vi "OFBS_MainFunction.vi"(6 "ReInitialize?":bool, 8 "Stop ButtonRef in":refnum<vi>, 9 "Results ListBox Ref":refnum<vi>, 10 "Fitness Chart Ref in":refnum<vi>, 11 "OFBS metaparameters in":T1={"Training Data Path"=path "", "Test Data Path"=path "", "True Labels for Test Trials"=path "", "Optimization Algorithm"=enum."Genetic algorithm", "ClassifierType"=enum."Multilayer perceptron", "GA Parameters"={"Population size"=100, "Generations no."=500, "Significant digits"=4, "Crossover probabality"=0.85, "Mutation mode"=enum."one-point, fixed rate", "Use Gray code?"=FALSE, "Mutation rate"=0.05, "Min mutation rate"=0.0005, "Max mutation rate"=0.25, "Reproduction plan"=enum."Steady-state-replace-worst", "Elitism"=FALSE, "Fmax"=1}, "PSO Parameters"={"Swarm size"=50, "Generations no."=10, "Cognitive coeff a1"=2.05, "Social coeff a2"=2.05, "Min inertia weight"=0.4, "Max inertia weight "=0.9, "Fmax"=0}, "Number of Channels"=0, "Use equal number of trials?"=FALSE, "Classifier Metaparameter"=0.0, "ClassifierQualityMeasure"=enum."Accuracy"} {"Classifier Metaparameter" min=0.0 max=100.0 step=0.1 format="%#_2g"; "PSO Parameters"."Generations no." min=1; "PSO Parameters"."Swarm size" min=1; "GA Parameters"."Max mutation rate" min=0.0 max=1.0; "GA Parameters"."Min mutation rate" min=0.0 max=1.0; "GA Parameters"."Mutation rate" min=0.0 max=1.0; "GA Parameters"."Crossover probabality" min=0.0 max=1.0; "GA Parameters"."Significant digits" min=1; "GA Parameters"."Generations no." min=1; "GA Parameters"."Population size" min=1}) -> (0 "Results dbl":dbl[](array[numeric]), 3 "Results str":string[](array[string]))   [LabVIEW 2016, in "Optimal Frequency Bands Search.lvlib"]
doc: "Главный виртуальный прибор проекта. Реализует графический интерфейс взаимодействия с пользователем."
uses:
  Optimal Frequency Bands Search.lvlib
  _vlib/OFBS_metaParameters.ctl
  _vlib/OFBS_AlgorithmTypes.ctl
  4. Accuracy Assessment for EEG Classification/_vlib/CU_ClassifierTypes.ctl
  GA_core/GA_tParameters.ctl
  particle_swarm_opt/PSO_tParameters.ctl
  4. Accuracy Assessment for EEG Classification/_vlib/CU_ClassifierQualityMeasure.ctl
  _vlib/OFBS_AppStates.ctl
  _vlib/OptFreqBandsSearch.lvclass
  GA_core/GA_tFitness Function.ctl
  GA_core/GA_tPopulation.ctl
  GA_core/GA_tSolution progress.ctl
  particle_swarm_opt/tFitness Function.ctl
  particle_swarm_opt/PSO_tPopulation.ctl
  particle_swarm_opt/PSO_tSolution progress.ctl
  GA_core/GeneticAlgorithm.lvlib
  particle_swarm_opt/ParticleSwarm.lvlib
  4. Accuracy Assessment for EEG Classification/Classifier.lvlib
panel:
  out "Solution":i32[][][](array[numeric])
  out "Accuracy":dbl caption="Приспособ-\nленность"
  out "Generation":i32 caption="Поколение"
  out "Trials of each class":i32[](array[numeric]) caption="Число проб \nкаждого класса"
  out "Reading File":path caption="Чтение файла"
  out "Progress":i32(slide) caption="Процесс чтения" min=0 max=320 scale=0.0..288.0
  out "Number of Trials":i32 caption="Число проб в файле"
  out "Application State":string caption="Состояние"
  # "This VI is a part of BCI Design library, http://www.ru-bci.org \nCopyright © 2020, Sotnikov Peter, All rights reserved. License: CC BY-NC 4.0"
  # "Fo"
  # "deltaF"
  # "Точность\nна тестовой\nвыборке"
  # "Точность\nна обучающей\nвыборке"
  # "Точность\nна контрол. \nвыборке"
  # "Sotnikov P (c), 2016"
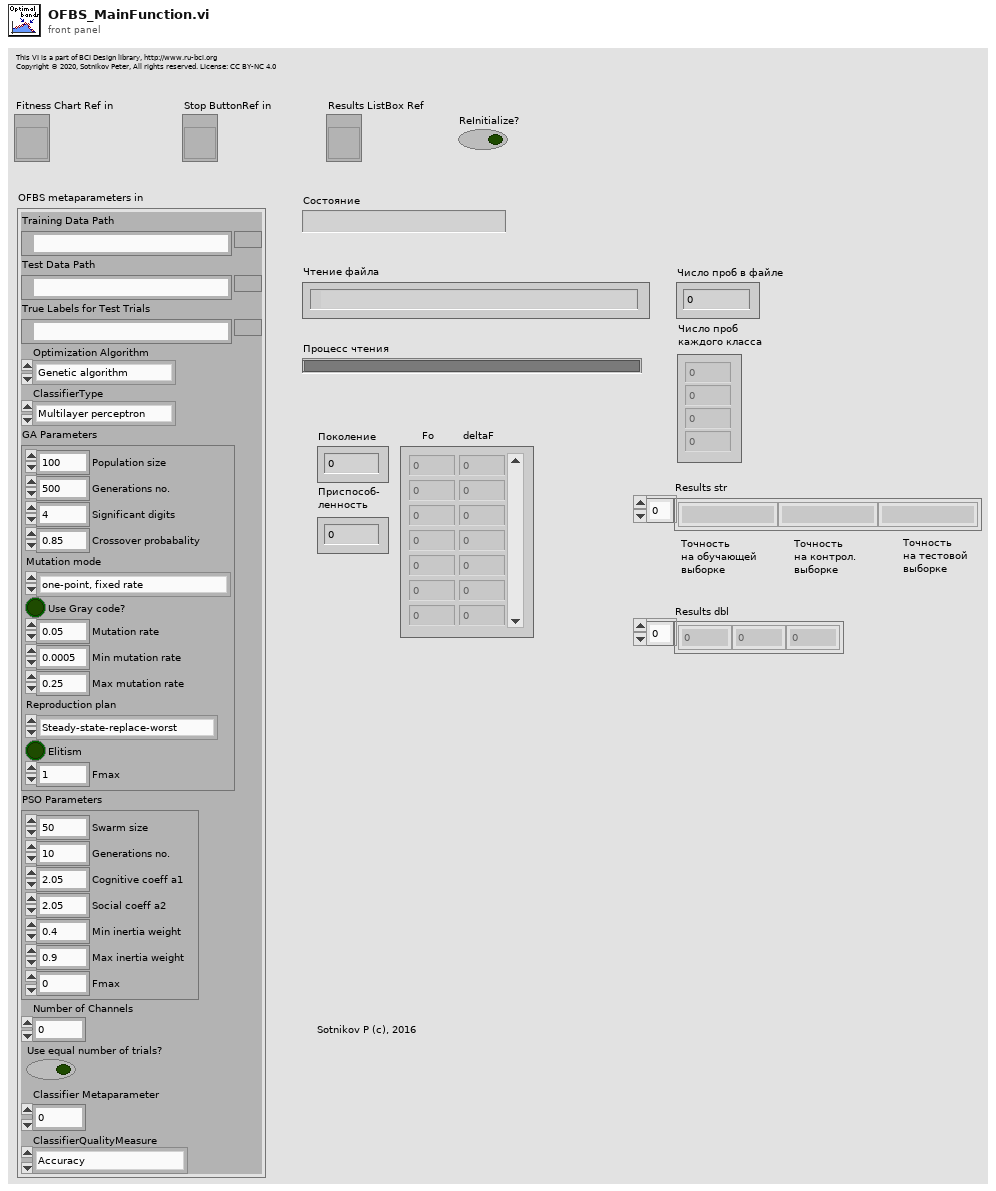
[diagram p1: front panel]
types:
  T1 = typedef "Optimal Frequency Bands Search.lvlib/OFBS_metaParameters.ctl" = cluster{"Training Data Path":path, "Test Data Path":path, "True Labels for Test Trials":path, "Optimization Algorithm":T2, "ClassifierType":T3, "GA Parameters":T4, "PSO Parameters":T5, "Number of Channels":i32, "Use equal number of trials?":bool, "Classifier Metaparameter":dbl, "ClassifierQualityMeasure":T6}
  T2 = typedef "Optimal Frequency Bands Search.lvlib/OFBS_AlgorithmTypes.ctl" = enum16{"Genetic algorithm", "Particle swarm optimization"}
  T3 = typedef "Classifier.lvlib/CU_ClassifierTypes.ctl" = enum16{"Multilayer perceptron", "k NN Classifier", "SVM Committee", "Mahalanobis distance", "SVM Classifier"}
  T4 = typedef "Optimal Frequency Bands Search.lvlib/GeneticAlgorithm.lvlib/GA_tParameters.ctl" = cluster{"Population size":i32, "Generations no.":i32, "Significant digits":i32, "Crossover probabality":dbl, "Mutation mode":enum16{"one-point, fixed rate", "one-point, fitness-adjustable rate", "one-point, distance-adjustable rate"}, "Use Gray code?":bool, "Mutation rate":dbl, "Min mutation rate":dbl, "Max mutation rate":dbl, "Reproduction plan":enum16{"Full generational replacement", "Steady-state-replace-random", "Steady-state-replace-worst"}, "Elitism":bool, "Fmax":i32}
  T5 = typedef "Optimal Frequency Bands Search.lvlib/ParticleSwarm.lvlib/PSO_tParameters.ctl" = cluster{"Swarm size":i32, "Generations no.":i32, "Cognitive coeff a1":dbl, "Social coeff a2":dbl, "Min inertia weight":dbl, "Max inertia weight ":dbl, "Fmax":i32}
  T6 = typedef "Classifier.lvlib/CU_ClassifierQualityMeasure.ctl" = enum16{"Accuracy", "Cohen's kappa"}
  T7 = typedef "Optimal Frequency Bands Search.lvlib/OFBS_AppStates.ctl" = enum16{"Initialize", "ReadTrainData", "ReadTestData", "StartOptimization", "Optimization_GA", "Optimization_PSO", "Stop"}
  T8 = typedef "Optimal Frequency Bands Search.lvlib/GeneticAlgorithm.lvlib/GA_tFitness Function.ctl" = refnum<vi>
  T9 = typedef "Optimal Frequency Bands Search.lvlib/ParticleSwarm.lvlib/tFitness Function.ctl" = refnum<vi>
  T10 = cluster{"Training Data Path":path, "Test Data Path":path, "True Labels for Test Trials":path}
  T11 = cluster{"Number of Trials":refnum<vi>, "Progress":refnum<vi>}
  T12 = typedef "Optimal Frequency Bands Search.lvlib/GeneticAlgorithm.lvlib/GA_tSolution progress.ctl" = cluster{"Solution":i32[], "Fitness":dbl, "Mutation rate":dbl, "Generation":i32}
  T13 = typedef "Optimal Frequency Bands Search.lvlib/GeneticAlgorithm.lvlib/GA_tPopulation.ctl" = cluster{"Population":i32[][], "Fitnesses":dbl[], "Sorted indices":i32[], "Ranks":i32[]}
  T14 = cluster{"Accuracy":refnum<vi>, "Generation":refnum<vi>, "Solution":refnum<vi>, "Fitness Chart Ref in":refnum<vi>}
  T15 = typedef "Optimal Frequency Bands Search.lvlib/ParticleSwarm.lvlib/PSO_tSolution progress.ctl" = cluster{"Solution":i32[], "Fitness":dbl, "Inertia":dbl, "Generation":i32}
  T16 = typedef "Optimal Frequency Bands Search.lvlib/ParticleSwarm.lvlib/PSO_tPopulation.ctl" = cluster{"Particle Coordinates":i32[][], "Fitnesses":dbl[], "Sorted indices":i32[], "Pbest Fitnesses":dbl[], "Pbest Particle Coordinates":i32[][], "Previous Velocity":dbl[][]}
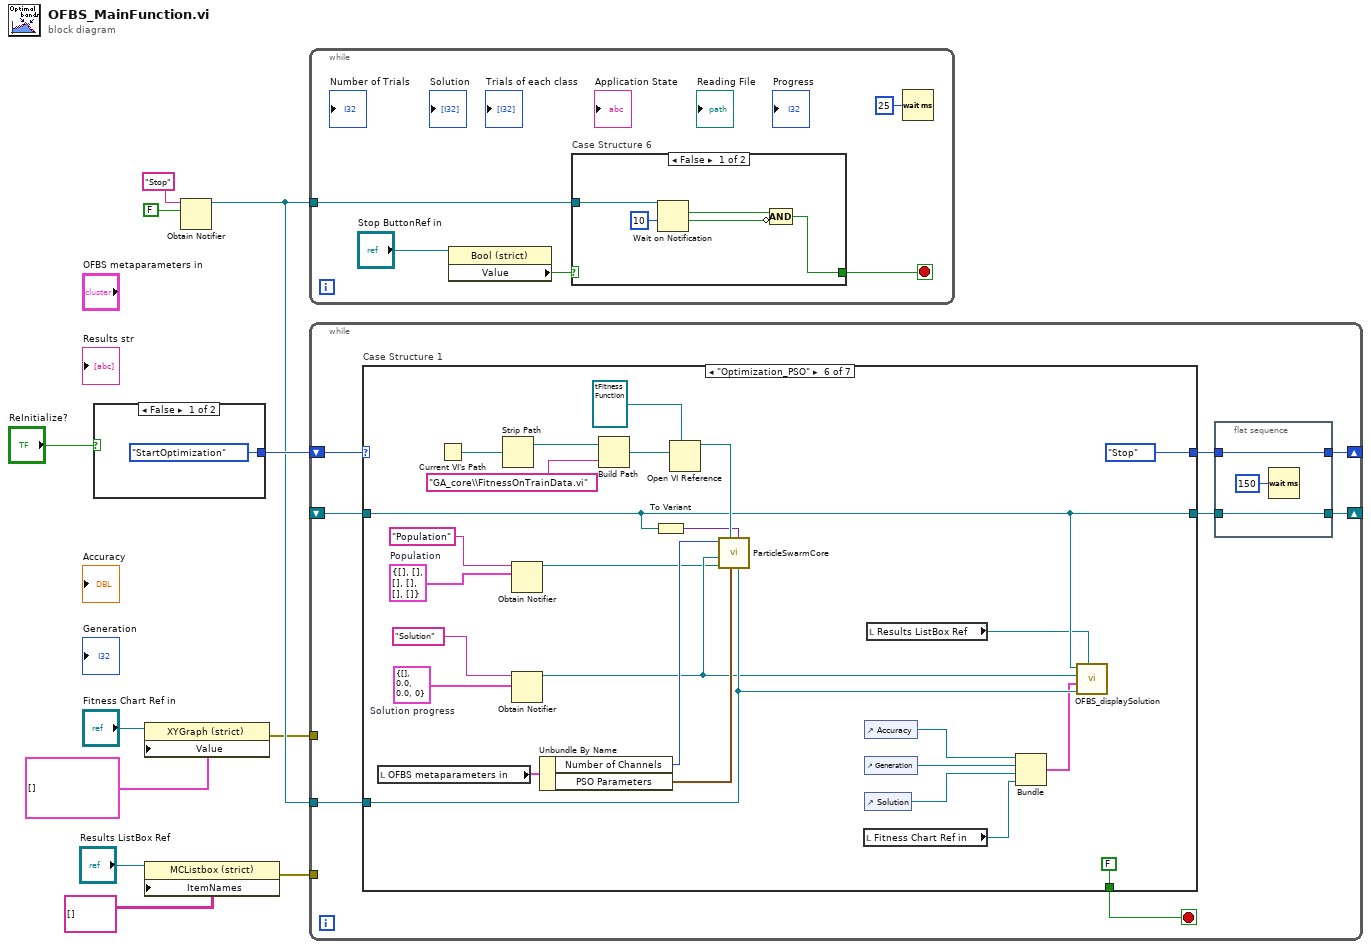
[diagram p0: block diagram]
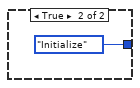
[diagram p2: hidden frame]
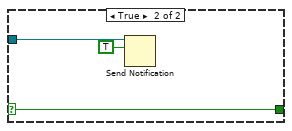
[diagram p3: hidden frame]
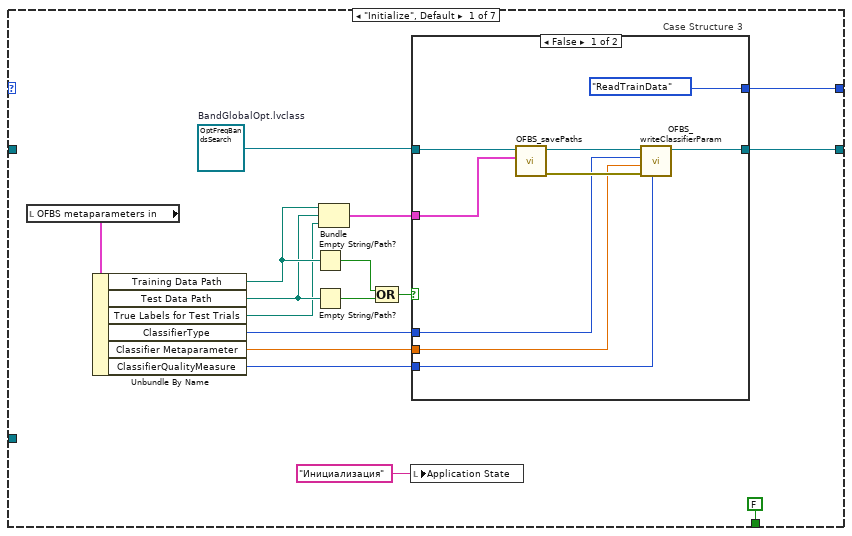
[diagram p4: hidden frame]
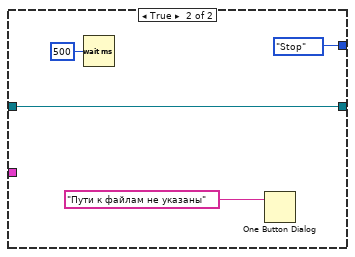
[diagram p5: hidden frame]
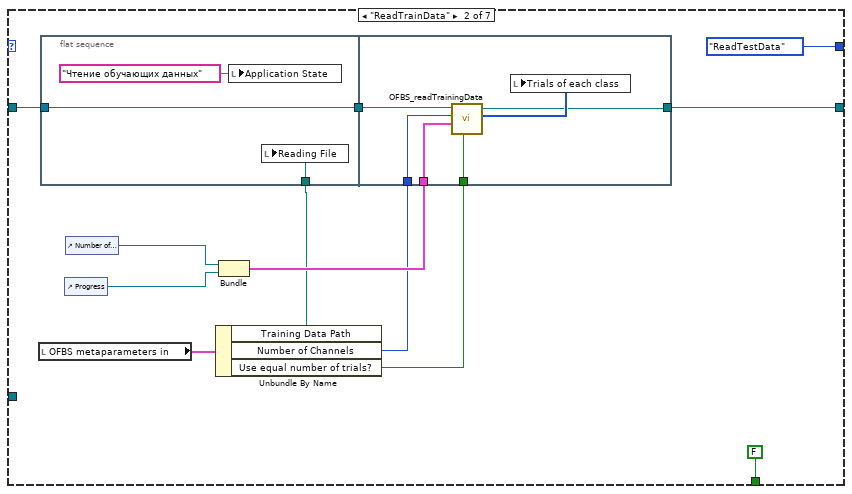
[diagram p6: hidden frame]
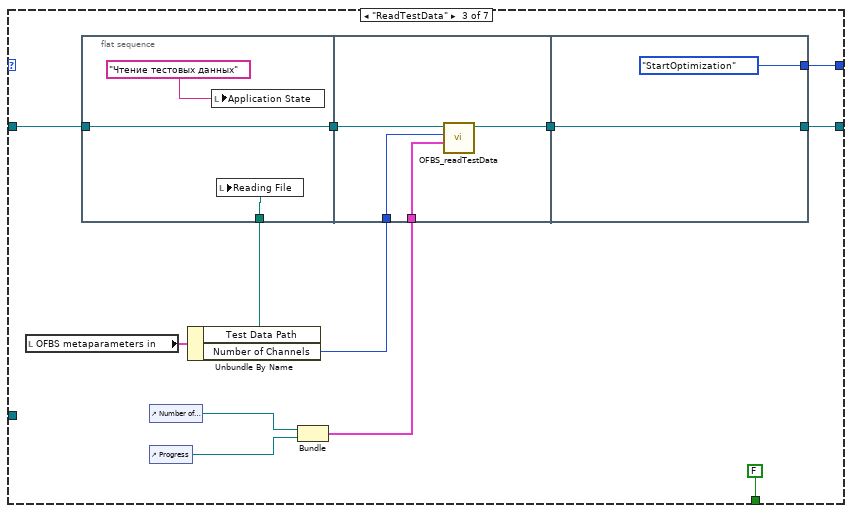
[diagram p7: hidden frame]
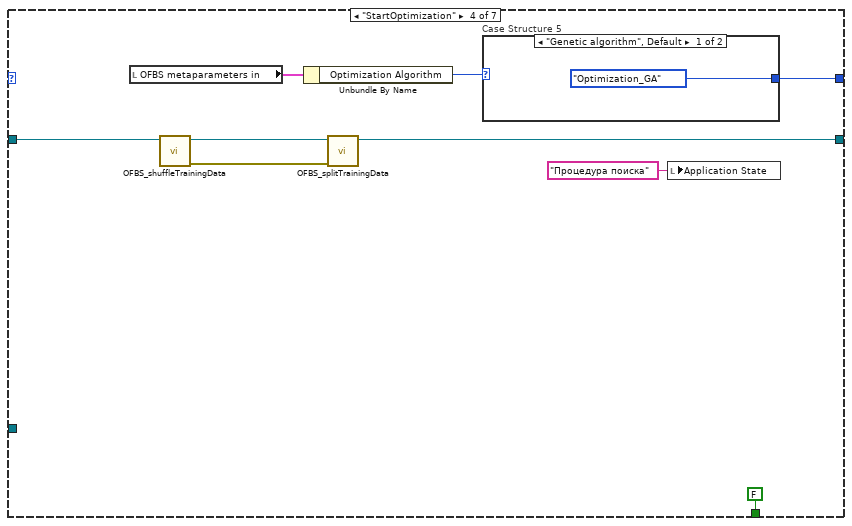
[diagram p8: hidden frame]
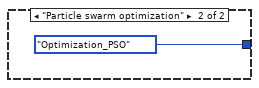
[diagram p9: hidden frame]
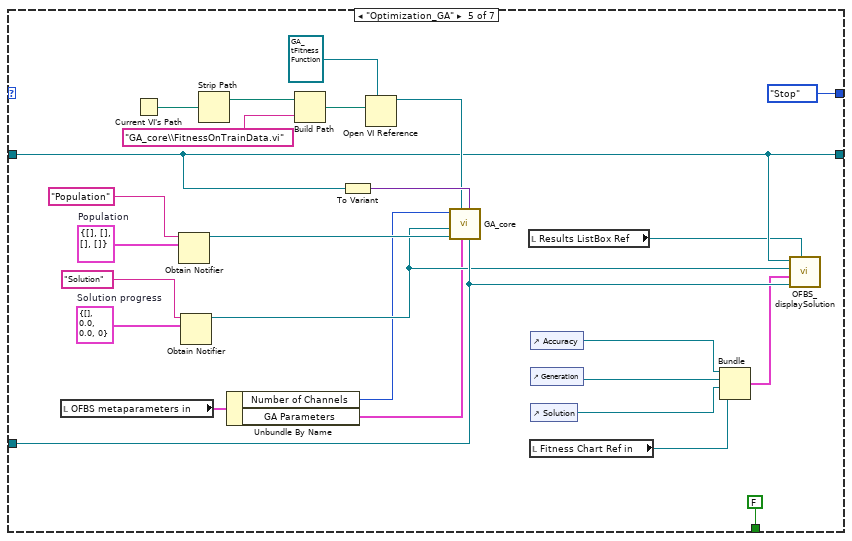
[diagram p10: hidden frame]
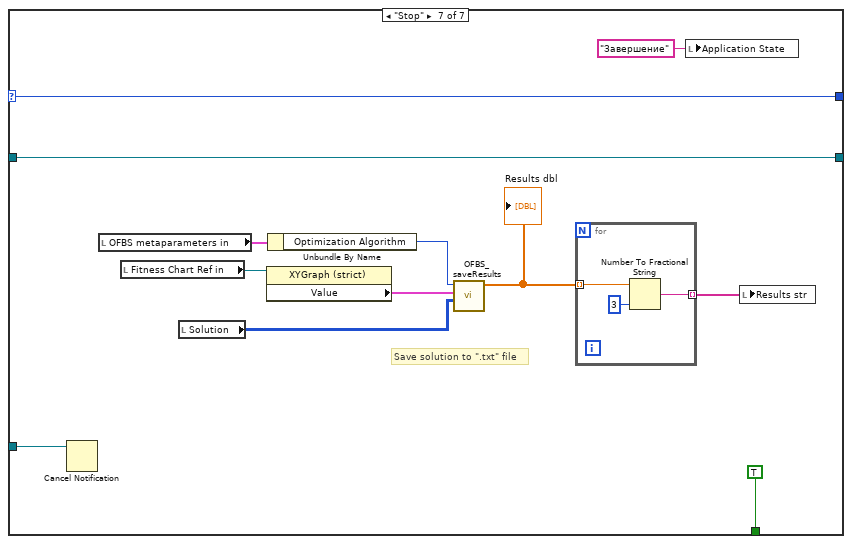
[diagram p11: hidden frame]
diagram:
  n1 = case shown="False" "ReInitialize?" {
    tunnel: [OFBS_AppStates."StartOptimization" ("BGO_AppStates") OFBS_AppStates."Initialize" ("BGO_AppStates")] -> w11
    frame False {
    }
    frame True {
    }
  }
  n2 = property class="XYGraph (strict)"(reference="Fitness Chart Ref in", "Value"=cluster{i32[], dbl[]}[] []) -> (error out=w6:errorcluster)  [unwired: 1 in, 1 out]
  n3 = property class="MCListbox (strict)"(reference="Results ListBox Ref", "ItemNames"=string[][] [] ("Item Names")) -> (error out=w3:errorcluster)  [unwired: 1 in, 1 out]
  n4 = Obtain Notifier(name (unnamed)="Stop", notification data type=FALSE) -> (notifier out=w8:refnum<notifier>)  [unwired: 2 in, 2 out]
  n5 = while {
    tunnel: w8 -> [w17]
    stop <- w16 stop-if-true
    n6 = property class="Bool (strict)"(reference="Stop ButtonRef in") -> ("Value"=w14:bool)  [unwired: 1 in, 2 out]
    n7 = case "Case Structure 6" shown="False" w14 {
      selector: w14 -> [_ w24]
      tunnel: w17 -> [w20 w26]
      tunnel: [w19 w24] -> w16
      frame False {
        n8 = Wait on Notification(notifier=w20, timeout in ms (-1)=10) -> (notification=w22:bool, timed out?=w23:bool)  [unwired: 2 in, 2 out]
        n9 = Compound Arithmetic op=AND(w22, invert w23) -> (w19:bool)
      }
      frame True {
        n10 = Send Notification(notification=TRUE, notifier=w26) -> ()  [unwired: 1 in, 2 out]
      }
    }
    n11 = Wait (ms)(milliseconds to wait=u32 25) -> ()  [unwired: 1 out]
  }
  n12 = while {
    shift-right: [w29] -> _
    shift-left: w11 -> [w34]
    shift-right: [w27] -> _
    shift-left: _ -> [w33]
    tunnel: w8 -> [w32]
    tunnel: w6 -> [_]
    tunnel: w3 -> [_]
    stop <- w31 stop-if-true
    n13 = case "Case Structure 1" shown="\"Optimization_PSO\"" w34 {
      selector: w34 -> [_ _ _ _ _ _ w183]
      tunnel: [FALSE ("Stop") FALSE FALSE FALSE ("Stop") FALSE FALSE TRUE] -> w31
      tunnel: [w53 OFBS_AppStates."ReadTestData" ("BGO_AppStates") w91 w117 OFBS_AppStates."Stop" ("BGO_AppStates") OFBS_AppStates."Stop" ("BGO_AppStates") w183] -> w30
      tunnel: w33 -> [_ w74 w99 w111 w127 w159 w182]
      tunnel: [w52 w73 w97 w112 w127 w159 w182] -> w28
      tunnel: w32 -> [_ _ _ _ w132 w158 w176]
      frame "Initialize", Default {
        w40 = refnum<class "OptFreqBandsSearch.lvclass"> refnum  # BandGlobalOpt.lvclass
        n14 = local read "OFBS metaparameters in"() -> (w46:T1)
        n15 = Unbundle By Name(w46) -> ("Training Data Path"=w45:path, "Test Data Path"=w44:path, "True Labels for Test Trials"=w43:path, "ClassifierType"=w42:T3, "Classifier Metaparameter"=w39:dbl, "ClassifierQualityMeasure"=w38:T6)
        n16 = Empty String/Path?(string/path=w45) -> (empty?=w50:bool)
        n17 = Empty String/Path?(string/path=w44) -> (empty?=w49:bool)
        n18 = Bundle("Training Data Path"=w45, "Test Data Path"=w44, "True Labels for Test Trials"=w43) -> (w47:T10)  [unwired: 1 in]
        n19 = Compound Arithmetic op=OR(w50, w49) -> (w48:bool)
        n20 = local write "Application State"("Инициализация" ("Application State")) -> ()
        n21 = case "Case Structure 3" shown="False" w48 {
          tunnel: [OFBS_AppStates."ReadTrainData" ("BGO_AppStates") OFBS_AppStates."Stop" ("BGO_AppStates")] -> w53
          tunnel: w40 -> [w61 w65]
          tunnel: [w57 w65] -> w52
          tunnel: w47 -> [w60 _]
          tunnel: w42 -> [w56 _]
          tunnel: w39 -> [w55 _]
          tunnel: w38 -> [w54 _]
          frame False {
            n22 = call "OFBS_savePaths.vi"("Paths"=w60, "BandGlobalOpt in"=w61) -> ("error out"=w58:errorcluster, "BandGlobalOpt out"=w59:refnum<class "OptFreqBandsSearch.lvclass">)  [unwired: 8 in]
            n23 = call-dynamic "OFBS_writeClassifierParam.vi"("Quality Measure in"=w54, "error in (no error)"=w58, "Metaparameter in"=w55, "Classifier Type in"=w56, "OptFreqBandsSearch in"=w59) -> ("OptFreqBandsSearch out"=w57:refnum<class "OptFreqBandsSearch.lvclass">)  [unwired: 5 in, 1 out]
          }
          frame True {
            n24 = Wait (ms)(milliseconds to wait=u32 500) -> ()  [unwired: 1 out]
            n25 = One Button Dialog(message="Пути к файлам не указаны" ("Application State")) -> ()  [unwired: 1 in, 1 out]
          }
        }
      }
      frame "ReadTrainData" {
        n26 = local read "OFBS metaparameters in"() -> (w70:T1)
        n27 = flat-sequence {
          tunnel: w74 -> [w81]
          tunnel: [w81] -> w72
          tunnel: w68 -> [w79]
          tunnel: [w82] -> w73
          tunnel: w71 -> [w86]
          tunnel: w72 -> [w87]
          tunnel: w69 -> [w85]
          tunnel: w67 -> [w84]
          frame #0 {
            n28 = local write "Application State"("Чтение обучающих данных" ("Application State")) -> ()
            n29 = local write "Reading File"(w79) -> ()
          }
          frame #1 {
            n30 = call "OFBS_readTrainingData.vi"("Use equal number of trials?"=w84, "ControlRefs"=w86, "NumberOfChannels"=w85, "OFBS class in"=w87) -> ("Num of Trials of each Class"=w83:i32[], "OFBS class out"=w82:refnum<class "OptFreqBandsSearch.lvclass">)  [unwired: 5 in, 1 out]
            n31 = local write "Trials of each class"(w83) -> ()
          }
        }
        n32 = control-ref of="Progress"() -> (w78:refnum<vi>)
        n33 = control-ref of="Number of Trials"() -> (w77:refnum<vi>)
        n34 = Unbundle By Name(w70) -> ("Training Data Path"=w68:path, "Number of Channels"=w69:i32, "Use equal number of trials?"=w67:bool)
        n35 = Bundle("Number of Trials"=w77, "Progress"=w78) -> (w71:T11)  [unwired: 1 in]
      }
      frame "ReadTestData" {
        n36 = local read "OFBS metaparameters in"() -> (w90:T1)
        n37 = flat-sequence {
          tunnel: w99 -> [w102]
          tunnel: [w102] -> w93
          tunnel: w88 -> [w100]
          tunnel: w95 -> [w104]
          tunnel: w89 -> [w103]
          tunnel: w93 -> [w106]
          tunnel: [w105] -> w92
          tunnel: [w108] -> w97
          tunnel: w92 -> [w108]
          tunnel: [OFBS_AppStates."StartOptimization" ("BGO_AppStates")] -> w91
          frame #0 {
            n38 = local write "Application State"("Чтение тестовых данных" ("Application State")) -> ()
            n39 = local write "Reading File"(w100) -> ()
          }
          frame #1 {
            n40 = call "OFBS_readTestData.vi"("ControlRefs"=w104, "NumberOfChannels"=w103, "OFBS class in"=w106) -> ("OFBS class out"=w105:refnum<class "OptFreqBandsSearch.lvclass">)  [unwired: 7 in, 1 out]
          }
          frame #2 {
          }
        }
        n41 = control-ref of="Number of Trials"() -> (w94:refnum<vi>)
        n42 = control-ref of="Progress"() -> (w98:refnum<vi>)
        n43 = Unbundle By Name(w90) -> ("Test Data Path"=w88:path, "Number of Channels"=w89:i32)
        n44 = Bundle("Number of Trials"=w94, "Progress"=w98) -> (w95:T11)  [unwired: 1 in]
      }
      frame "StartOptimization" {
        n45 = local read "OFBS metaparameters in"() -> (w115:T1)
        n46 = call "OFBS_shuffleTrainingData.vi"("OptFreqBandsSearch in"=w111) -> ("error out"=w109:errorcluster, "OptFreqBandsSearch out"=w110:refnum<class "OptFreqBandsSearch.lvclass">)  [unwired: 9 in]
        n47 = Unbundle By Name(w115) -> ("Optimization Algorithm"=w114:T2)
        n48 = call "OFBS_splitTrainingData.vi"("error in (no error)"=w109, "OFBS class in"=w110) -> ("OFBS class out"=w112:refnum<class "OptFreqBandsSearch.lvclass">)  [unwired: 6 in, 3 out]
        n49 = case "Case Structure 5" shown="\"Genetic algorithm\", Default" w114 {
          tunnel: [OFBS_AppStates."Optimization_GA" ("BGO_AppStates") OFBS_AppStates."Optimization_PSO" ("BGO_AppStates")] -> w117
          frame "Genetic algorithm", Default {
          }
          frame "Particle swarm optimization" {
          }
        }
        n50 = local write "Application State"("Процедура поиска" ("Application State")) -> ()
      }
      frame "Optimization_GA" {
        w135 = T12 {"Solution"=[], "Fitness"=0.0, "Mutation rate"=0.0, "Generation"=0}  # Solution progress
        w137 = T13 {"Population"=[], "Fitnesses"=[], "Sorted indices"=[], "Ranks"=[]}  # Population
        n51 = local read "OFBS metaparameters in"() -> (w124:T1)
        n52 = Current VI's Path() -> (path=w142:path)
        n53 = Obtain Notifier(name (unnamed)="Population", notification data type=w137) -> (notifier out=w133:refnum<notifier>)  [unwired: 2 in, 2 out]
        n54 = Obtain Notifier(name (unnamed)="Solution", notification data type=w135) -> (notifier out=w128:refnum<notifier>)  [unwired: 2 in, 2 out]
        n55 = Strip Path(path=w142) -> (stripped path=w141:path)  [unwired: 1 out]
        n56 = Unbundle By Name(w124) -> ("Number of Channels"=w123:i32, "GA Parameters"=w122:T4)
        n57 = Build Path(base path=w141, name or relative path="GA_core\\FitnessOnTrainData.vi") -> (appended path=w139:path)
        n58 = To Variant(anything=w127) -> (Variant=w143:variant)
        n59 = Open VI Reference(type specifier VI Refnum (for type only)=T8 refnum ("Fitness Function"), vi path=w139) -> (vi reference=w138:T8)  [unwired: 4 in, 1 out]
        n60 = call "GA_core.vi"("Stop notifier"=w132, "Fitness Function Data"=w143, "Parameters"=w122, "Fitness Function"=w138, "Population notifier"=w133, "Solution Progress notifier"=w128, "Phenotype size"=w123) -> ()  [unwired: 2 in, 3 out]
        n61 = local read "Results ListBox Ref"() -> (w120:refnum<vi>)
        n62 = local read "Fitness Chart Ref in"() -> (w121:refnum<vi>)
        n63 = control-ref of="Accuracy"() -> (w131:refnum<vi>)
        n64 = control-ref of="Generation"() -> (w130:refnum<vi>)
        n65 = control-ref of="Solution"() -> (w129:refnum<vi>)
        n66 = Bundle("Accuracy"=w131, "Generation"=w130, "Solution"=w129, "Fitness Chart Ref in"=w121) -> (w126:T14)  [unwired: 1 in]
        n67 = call "OFBS_displaySolution.vi"("Results ListBox Ref"=w120, "Stop Notifier In"=w132, "Control Refs"=w126, "Solution notifier"=w128, "BandGlobalOpt.lvclass"=w127) -> ()  [unwired: 7 in]
      }
      frame "Optimization_PSO" {
        w161 = T15 {"Solution"=[], "Fitness"=0.0, "Inertia"=0.0, "Generation"=0}  # Solution progress
        w163 = T16 {"Particle Coordinates"=[], "Fitnesses"=[], "Sorted indices"=[], "Pbest Fitnesses"=[], "Pbest Particle Coordinates"=[], "Previous Velocity"=[]}  # Population
        n68 = local read "OFBS metaparameters in"() -> (w152:T1)
        n69 = Current VI's Path() -> (path=w171:path)
        n70 = Strip Path(path=w171) -> (stripped path=w170:path)  [unwired: 1 out]
        n71 = Obtain Notifier(name (unnamed)="Population", notification data type=w163) -> (notifier out=w148:refnum<notifier>)  [unwired: 2 in, 2 out]
        n72 = Obtain Notifier(name (unnamed)="Solution", notification data type=w161) -> (notifier out=w149:refnum<notifier>)  [unwired: 2 in, 2 out]
        n73 = Unbundle By Name(w152) -> ("Number of Channels"=w151:i32, "PSO Parameters"=w150:T5)
        n74 = Build Path(base path=w170, name or relative path="GA_core\\FitnessOnTrainData.vi") -> (appended path=w168:path)
        n75 = To Variant(anything=w159) -> (Variant=w164:variant)
        n76 = Open VI Reference(type specifier VI Refnum (for type only)=T9 refnum ("Fitness Function"), vi path=w168) -> (vi reference=w166:T9)  [unwired: 4 in, 1 out]
        n77 = call "ParticleSwarmCore.vi"("Stop notifier"=w158, "Fitness Function Data"=w164, "Parameters"=w150, "Fitness Function"=w166, "Population notifier"=w148, "Solution Progress notifier"=w149, "Phenotype size"=w151) -> ()  [unwired: 2 in, 3 out]
        n78 = local read "Fitness Chart Ref in"() -> (w147:refnum<vi>)
        n79 = control-ref of="Accuracy"() -> (w155:refnum<vi>)
        n80 = control-ref of="Generation"() -> (w156:refnum<vi>)
        n81 = control-ref of="Solution"() -> (w157:refnum<vi>)
        n82 = local read "Results ListBox Ref"() -> (w146:refnum<vi>)
        n83 = Bundle("Accuracy"=w155, "Generation"=w156, "Solution"=w157, "Fitness Chart Ref in"=w147) -> (w154:T14)  [unwired: 1 in]
        n84 = call "OFBS_displaySolution.vi"("Results ListBox Ref"=w146, "Stop Notifier In"=w158, "Control Refs"=w154, "Solution notifier"=w149, "BandGlobalOpt.lvclass"=w159) -> ()  [unwired: 7 in]
      }
      frame "Stop" {
        # "Save solution to \".txt\" file"
        n85 = Cancel Notification(0:w176) -> ()  [unwired: 1 in, 3 out]
        n86 = local read "OFBS metaparameters in"() -> (w178:T1)
        n87 = local read "Fitness Chart Ref in"() -> (w175:refnum<vi>)
        n88 = local read "Solution"() -> (w179:i32[][][])
        n89 = property class="XYGraph (strict)"(reference=w175) -> ("Value"=w174:cluster{i32[], dbl[]}[])  [unwired: 1 in, 2 out]
        n90 = Unbundle By Name(w178) -> ("Optimization Algorithm"=w177:T2)
        n91 = call "OFBS_saveResults.vi"("Solution"=w179, "Accuracy Chart"=w174, "Optimization Algorithm"=w177) -> ("Results out"=w173:dbl[])  [unwired: 7 in, 1 out]
        "Results dbl" <- w173
        n92 = for {
          tunnel: w173 -> [w186] mode=indexing
          tunnel: [w184] -> w172 mode=indexing
          n93 = Number To Fractional String(number=w186, precision (6)=i16 3) -> (F-format string=w184:string)  [unwired: 2 in]
        }
        n94 = local write "Application State"("Завершение" ("Application State")) -> ()
        n95 = local write "Results str"(w172) -> ()
      }
    }
    n96 = flat-sequence {
      tunnel: w30 -> [w37]
      tunnel: [w37] -> w29
      tunnel: w28 -> [w36]
      tunnel: [w36] -> w27
      frame #0 {
        n97 = Wait (ms)(milliseconds to wait=u32 150) -> ()  [unwired: 1 out]
      }
    }
  }
